vi "Check Dependencies.vi"(10 "Variant":variant) -> (0 "error out":errorcluster)   [LabVIEW 2011, in "LVH-Leap.lvlib"]
uses:
  vi.lib/LabVIEW Hacker/Leap/LVH-Leap.lvlib
  <vilib>/LabVIEW Hacker/LVH-Toolbox/Installer Tools/Installer Tools.lvlib
  <vilib>/LabVIEW Hacker/LVH-Toolbox/Common/LVH-Common.lvlib
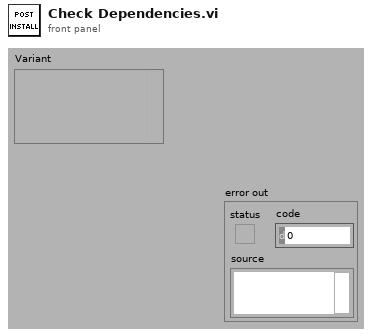
[diagram p1: front panel]
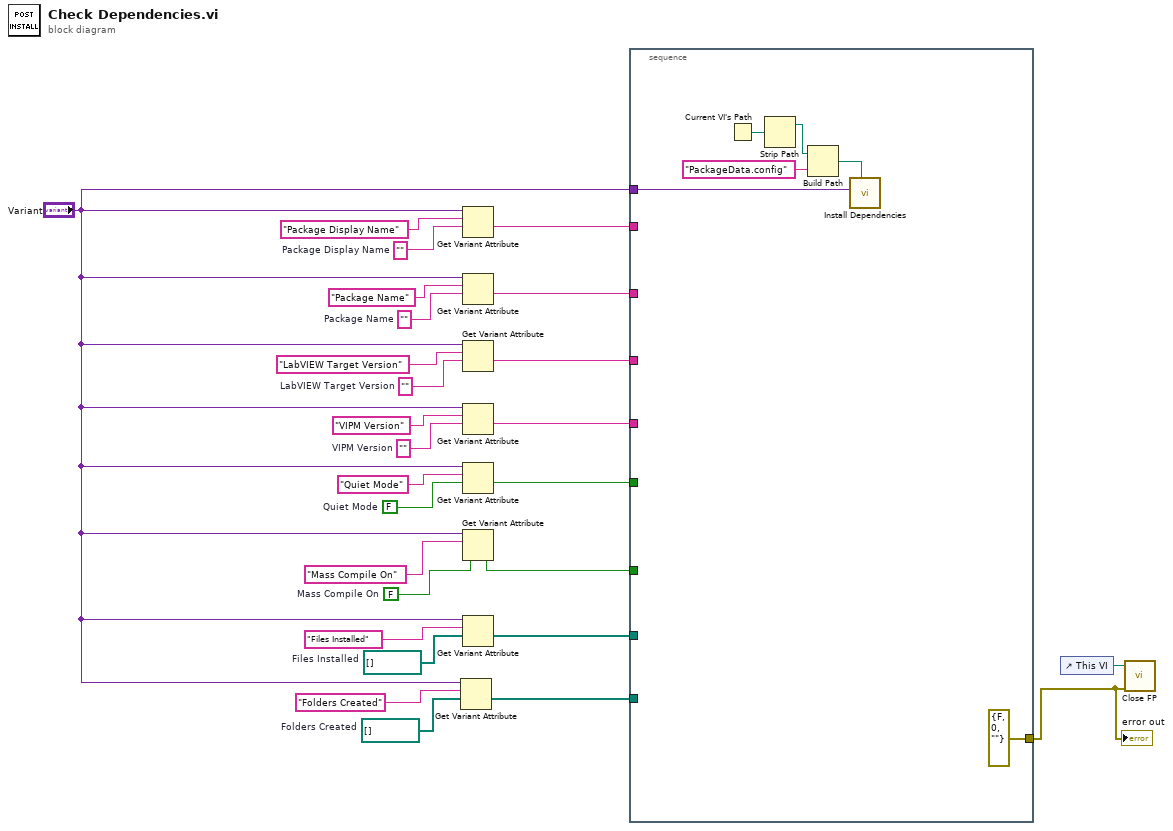
[diagram p0: block diagram]
diagram:
  w4 = path[] []  # Folders Created
  w5 = path[] []  # Files Installed
  w10 = FALSE  # Mass Compile On
  w11 = ""  # Package Display Name
  w18 = FALSE  # Quiet Mode
  w21 = ""  # VIPM Version
  w23 = ""  # LabVIEW Target Version
  w25 = ""  # Package Name
  n1 = Get Variant Attribute(Variant="Variant", name="Folders Created", default value (empty Variant)=w4) -> (value=w8:path[])  [unwired: 1 in, 3 out]
  n2 = Get Variant Attribute(Variant="Variant", name="Package Display Name", default value (empty Variant)=w11) -> (value=w17:string)  [unwired: 1 in, 3 out]
  n3 = Get Variant Attribute(Variant="Variant", name="Package Name", default value (empty Variant)=w25) -> (value=w16:string)  [unwired: 1 in, 3 out]
  n4 = Get Variant Attribute(Variant="Variant", name="LabVIEW Target Version", default value (empty Variant)=w23) -> (value=w15:string)  [unwired: 1 in, 3 out]
  n5 = Get Variant Attribute(Variant="Variant", name="VIPM Version", default value (empty Variant)=w21) -> (value=w14:string)  [unwired: 1 in, 3 out]
  n6 = Get Variant Attribute(Variant="Variant", name="Quiet Mode", default value (empty Variant)=w18) -> (value=w13:bool)  [unwired: 1 in, 3 out]
  n7 = Get Variant Attribute(Variant="Variant", name="Mass Compile On", default value (empty Variant)=w10) -> (value=w12:bool)  [unwired: 1 in, 3 out]
  n8 = Get Variant Attribute(Variant="Variant", name="Files Installed", default value (empty Variant)=w5) -> (value=w7:path[])  [unwired: 1 in, 3 out]
  n9 = stacked-sequence {
    tunnel: w17 -> [_]
    tunnel: w16 -> [_]
    tunnel: w15 -> [_]
    tunnel: w14 -> [_]
    tunnel: w13 -> [_]
    tunnel: w12 -> [_]
    tunnel: w7 -> [_]
    tunnel: w8 -> [_]
    tunnel: "Variant" -> [w33]
    tunnel: [errorcluster {"status"=FALSE, "code"=0, "source"=""} ("error out")] -> w1
    frame #0 {
      n10 = Current VI's Path() -> (path=w31:path)
      n11 = Strip Path(path=w31) -> (stripped path=w30:path)  [unwired: 1 out]
      n12 = Build Path(base path=w30, name or relative path="PackageData.config") -> (appended path=w28:path)
      n13 = call <vilib>:"Install Dependencies.vi"("Stored Install Data"=w28, "Variant"=w33) -> ()  [unwired: 9 in, 1 out]
    }
  }
  "error out" <- w1
  n14 = control-ref of="This VI"() -> (w2:refnum<vi>)
  n15 = call <vilib>:"Close FP.vi"("Error In"=w1, "VI Ref"=w2) -> ()  [unwired: 9 in, 1 out]
